vi "Encoder_GetSetRefNum.vi"(8 "error in (no error)":errorcluster, 9 "menu":T6, 10 "refnum name":string, 11 "RobotEncoderRef":T5) -> (0 "error out":errorcluster, 2 "names":string[](array[string]), 3 "RobotEncoderRef Out":T5)   [LabVIEW 2013]
uses:
  <vilib>/Rock Robotics/WPI/Encoder/WPI_EncoderDevRef.ctl
  <vilib>/Rock Robotics/SystemInterfaces/Encoder/FPGA_EncoderIdx.ctl
  <vilib>/Rock Robotics/SystemInterfaces/Counter/FPGA_CounterCtrSystemIndex.ctl
  <vilib>/Rock Robotics/WPI/Encoder/WPI_EncoderType.ctl
  <vilib>/Rock Robotics/WPI/Utilities/Refnum Registry Operation.ctl
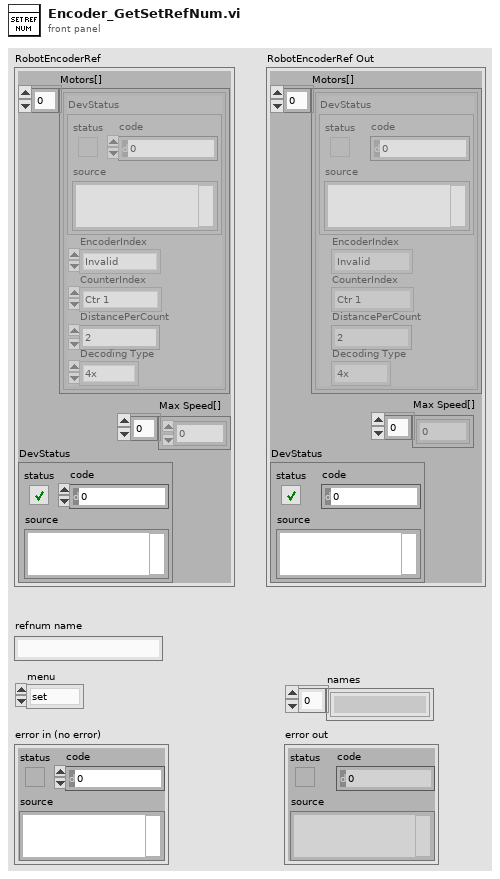
[diagram p1: front panel]
types:
  T1 = typedef "WPI_EncoderDevRef.ctl" = cluster{"DevStatus":errorcluster, "EncoderIndex":T2, "CounterIndex":T3, "DistancePerCount":dbl, "Decoding Type":T4}
  T2 = typedef "FPGA_EncoderIdx.ctl" = enum8{"Enc 0", "Enc 1", "Enc 2", "Enc 3", "Invalid"}
  T3 = typedef "FPGA_CounterCtrSystemIndex.ctl" = enum8{"Ctr 0", "Ctr 1", "Ctr 2", "Ctr 3", "Ctr 4", "Ctr 5", "Ctr 6", "Ctr 7", "Invalid"}
  T4 = typedef "WPI_EncoderType.ctl" = enum16{"1x", "2x", "4x"}
  T5 = cluster{"Motors[]":T1[], "DevStatus":errorcluster, "Max Speed[]":dbl[]}
  T6 = typedef "Refnum Registry Operation.ctl" = enum16{"set", "get", "delete", "get all names", "read name"}
  T7 = cluster{"Motors[]":T1[], "DevStatus":errorcluster, "Max Speed[]":dbl[]}[]
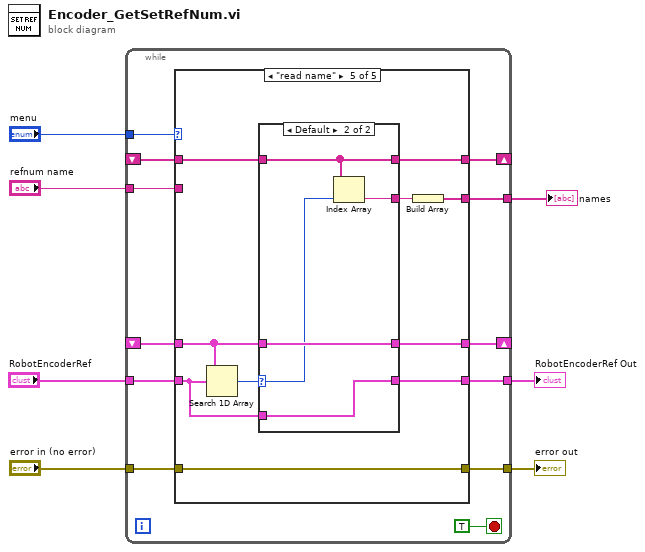
[diagram p0: block diagram]
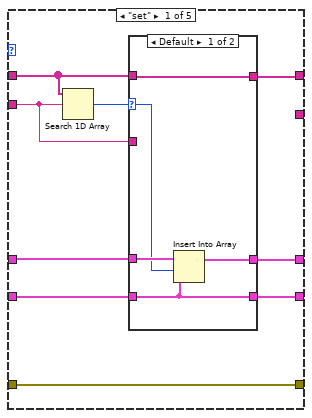
[diagram p2: hidden frame]
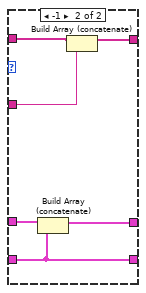
[diagram p3: hidden frame]
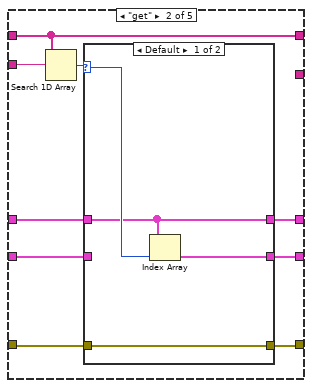
[diagram p4: hidden frame]
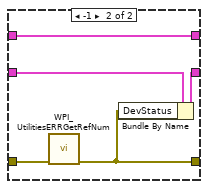
[diagram p5: hidden frame]
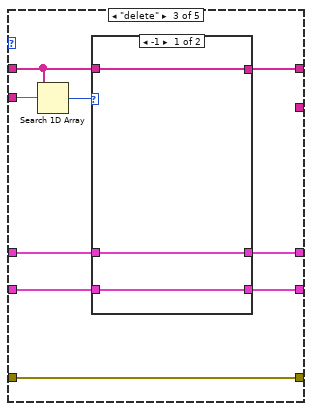
[diagram p6: hidden frame]
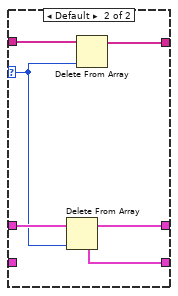
[diagram p7: hidden frame]
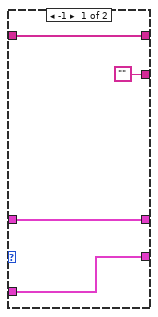
[diagram p9: hidden frame]
diagram:
  n1 = while {
    shift-right: [w17] -> _
    shift-left: _ -> [w16]
    shift-right: [w15] -> _
    shift-left: _ -> [w14]
    tunnel: "menu" -> [w18]
    tunnel: "refnum name" -> [w13]
    tunnel: [w12] -> w5
    tunnel: "error in (no error)" -> [w11]
    tunnel: [w10] -> w3
    tunnel: "RobotEncoderRef" -> [w9]
    tunnel: [w8] -> w1
    stop <- TRUE stop-if-true
    n2 = case shown="\"read name\"" w18 {
      tunnel: [w23 w44 w59 w79 w88] -> w17
      tunnel: w16 -> [w24 w44 w65 w79 w89]
      tunnel: [w26 w41 w62 w78 w85] -> w15
      tunnel: w14 -> [w27 w40 w63 w78 w81]
      tunnel: w13 -> [w22 w43 w66 _ _]
      tunnel: [w28 w47 w58 w76 w80] -> w12
      tunnel: w11 -> [w28 w48 w58 w76 w80]
      tunnel: [w20 w45 w61 w77 w84] -> w10
      tunnel: w9 -> [w25 w46 w64 w77 w82]
      tunnel: [_ _ _ w79 w87] -> w8
      frame "set" {
        n3 = Search 1D Array(1D array=w24, element=w22) -> (index of element=w21:i32)  [unwired: 1 in]
        n4 = case shown="Default" w21 {
          selector: w21 -> [w31 _]
          tunnel: w27 -> [w33 w39]
          tunnel: [w32 w38] -> w26
          tunnel: w25 -> [w29 w34]
          tunnel: w24 -> [w30 w37]
          tunnel: [w30 w36] -> w23
          tunnel: w22 -> [_ w35]
          tunnel: [w29 w34] -> w20
          frame Default {
            n5 = Insert Into Array(array=w33, index=w31, new element=w29) -> (w32:T7)
          }
          frame -1 {
            n6 = Build Array (concatenate)(w39, w34) -> (w38:T7)
            n7 = Build Array (concatenate)(w37, w35) -> (w36:string[])
          }
        }
      }
      frame "get" {
        n8 = Search 1D Array(1D array=w44, element=w43) -> (index of element=w42:i32)  [unwired: 1 in]
        n9 = case shown="Default" w42 {
          selector: w42 -> [w51 _]
          tunnel: w48 -> [w50 w57]
          tunnel: [w50 w56] -> w47
          tunnel: w46 -> [_ w55]
          tunnel: [w52 w54] -> w45
          tunnel: [w49 w53] -> w41
          tunnel: w40 -> [w49 w53]
          frame Default {
            n10 = Index Array(array=w49, index=w51) -> (element=w52:T5)
          }
          frame -1 {
            n11 = call <vilib>:"WPI_UtilitiesERRGetRefNum.vi"("error in (no error)"=w57) -> ("ERRGetRefNum"=w56:errorcluster)  [unwired: 10 out]
            n12 = Bundle By Name(cluster=w55, "DevStatus"=w56) -> (w54:T5)
          }
        }
      }
      frame "delete" {
        n13 = Search 1D Array(1D array=w65, element=w66) -> (index of element=w60:i32)  [unwired: 1 in]
        n14 = case shown="-1" w60 {
          selector: w60 -> [_ w71]
          tunnel: w65 -> [w69 w72]
          tunnel: w64 -> [w67 _]
          tunnel: w63 -> [w68 w75]
          tunnel: [w68 w74] -> w62
          tunnel: [w67 w73] -> w61
          tunnel: [w69 w70] -> w59
          frame -1 {
          }
          frame Default {
            n15 = Delete From Array(array=w75, index=w71) -> (deleted portion=w73:T5, array with subset deleted=w74:T7)  [unwired: 1 in]
            n16 = Delete From Array(array=w72, index=w71) -> (array with subset deleted=w70:string[])  [unwired: 1 in, 1 out]
          }
        }
      }
      frame "get all names", Default {
      }
      frame "read name" {
        n17 = Search 1D Array(1D array=w81, element=w82) -> (index of element=w83:i32)  [unwired: 1 in]
        n18 = case shown="Default" w83 {
          selector: w83 -> [_ w94]
          tunnel: w89 -> [w93 w98]
          tunnel: [w93 w98] -> w88
          tunnel: ["" w97] -> w86
          tunnel: w81 -> [w91 w96]
          tunnel: [w91 w96] -> w85
          tunnel: [w90 w95] -> w84
          tunnel: w82 -> [w90 w95]
          frame -1 {
          }
          frame Default {
            n19 = Index Array(array=w98, index=w94) -> (element=w97:string)
          }
        }
        n20 = Build Array(w86) -> (w87:string[])
      }
    }
  }
  "error out" <- w5
  "RobotEncoderRef Out" <- w3
  "names" <- w1
